vi "GV-GraphHoverAddYaxis.vi"(8 "error in (no error)":errorcluster, 9 "Pos":cluster{"x":i16, "y":i16}, 10 "Plot in":picture, 11 "Gviewer in":refnum<class "Gviewer.lvclass">) -> (0 "error out":errorcluster, 2 "Plot out":picture, 3 "Gviewer out":refnum<class "Gviewer.lvclass">)   [LabVIEW 2020, in "Sgraph_lib_V1.lvlib" / "Gviewer.lvclass"]
doc: "Andre Koelewijn, 27 April 2021\n\nMove legend over the graph area"
uses:
  Gviewer.lvclass
  <vilib>/Utility/miscctls.llb/LVPoint32TypeDef.ctl
  Gviewer.lvclass/Gviewer.ctl
panel:
  in  "Coords":T1
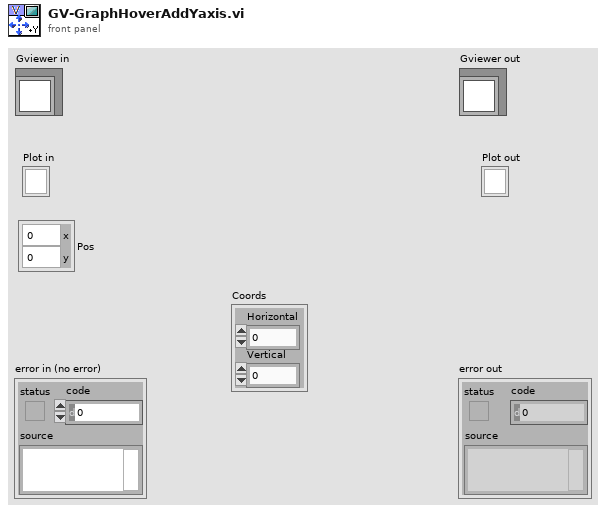
[diagram p1: front panel]
types:
  T1 = typedef "LVPoint32TypeDef.ctl" = cluster{"Horizontal":i32, "Vertical":i32}
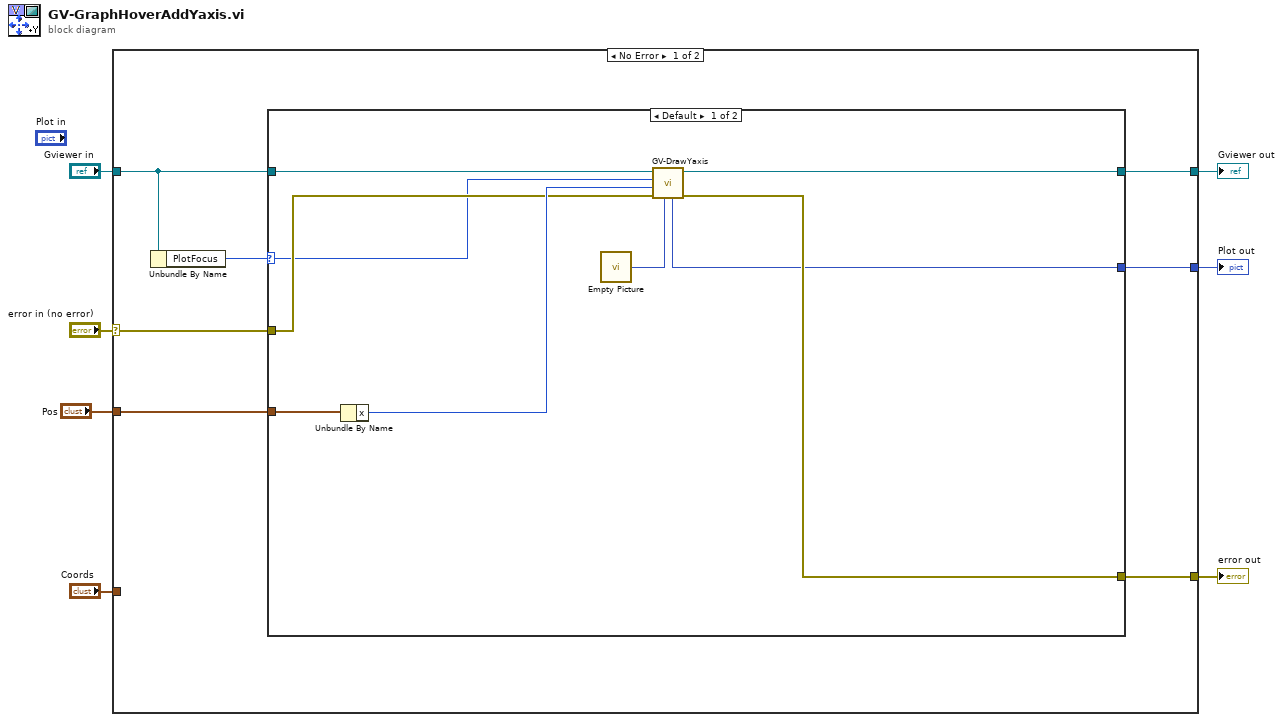
[diagram p0: block diagram]
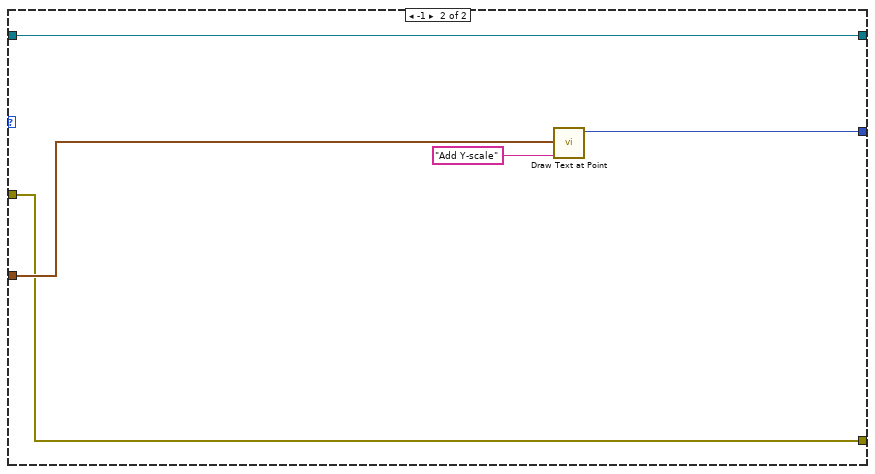
[diagram p2: hidden frame]
diagram:
  n1 = case shown="No Error" "error in (no error)" {
    selector: "error in (no error)" -> [w12 w30]
    tunnel: [w8 w30] -> w6
    tunnel: [w10 w29] -> w4
    tunnel: "Gviewer in" -> [w13 w29]
    tunnel: "Coords" -> [_ _]
    tunnel: [w9 _] -> w2
    tunnel: "Pos" -> [w11 _]
    frame No Error {
      n2 = Unbundle By Name(w13) -> ("PlotFocus"=w14:i32)
      n3 = case shown="Default" w14 {
        selector: w14 -> [w17 _]
        tunnel: [w15 w28] -> w9
        tunnel: w11 -> [w21 w26]
        tunnel: [w19 w25] -> w8
        tunnel: w12 -> [w18 w25]
        tunnel: w13 -> [w22 w24]
        tunnel: [w23 w24] -> w10
        frame Default {
          n4 = Unbundle By Name(w21) -> ("x"=w20:i16)
          n5 = call "Empty Picture"() -> ("empty picture"=w16:picture)
          n6 = call "GV-DrawYaxis.vi"("Picture IN"=w16, "error in (no error)"=w18, "X-position"=w20, "Plot"=w17, "Gviewer in"=w22) -> ("error out"=w19:errorcluster, "Gviewer out"=w23:refnum<class "Gviewer.lvclass">, "Picture OUT"=w15:picture)  [unwired: 4 in]
        }
        frame -1 {
          n7 = call <vilib>:"Draw Text at Point.vi"("text"="Add Y-scale", "origin"=w26) -> ("new picture"=w28:picture)  [unwired: 8 in, 1 out]
        }
      }
    }
    frame Error {
    }
  }
  "error out" <- w6
  "Gviewer out" <- w4
  "Plot out" <- w2
